vi "set_synth.vi"(0 "VISA resource name":refnum<visa-resource-name>, 1 "wfm?":bool, 3 "Arbitrary Waveform Name (\"ARB1\")":string="ARB1", 5 "Tot Synth Arr":dbl[](array[numeric]), 7 "error in (no error)":errorcluster, 9 "Enable Output (T: Enable)":bool=TRUE, 11 "Arbitrary Waveform Data":dbl[](array[numeric]), 12 "Trigger Synth":bool, 14 "Burst Count":i32=1) -> (4 "VISA resource name out":refnum<visa-resource-name>, 15 "error out":errorcluster)   [LabVIEW 2016]
uses:
  <instrlib>/Agilent 33XXX Series/Agilent 33XXX Series.lvlib
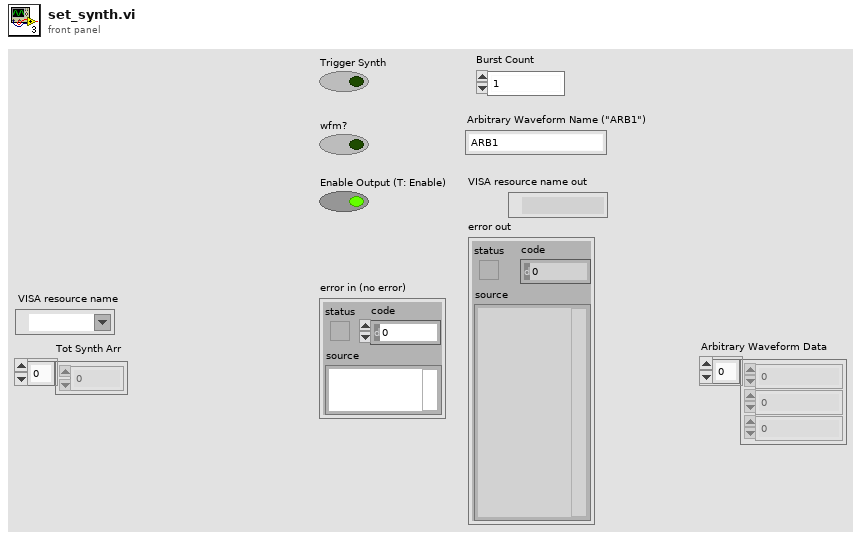
[diagram p1: front panel]
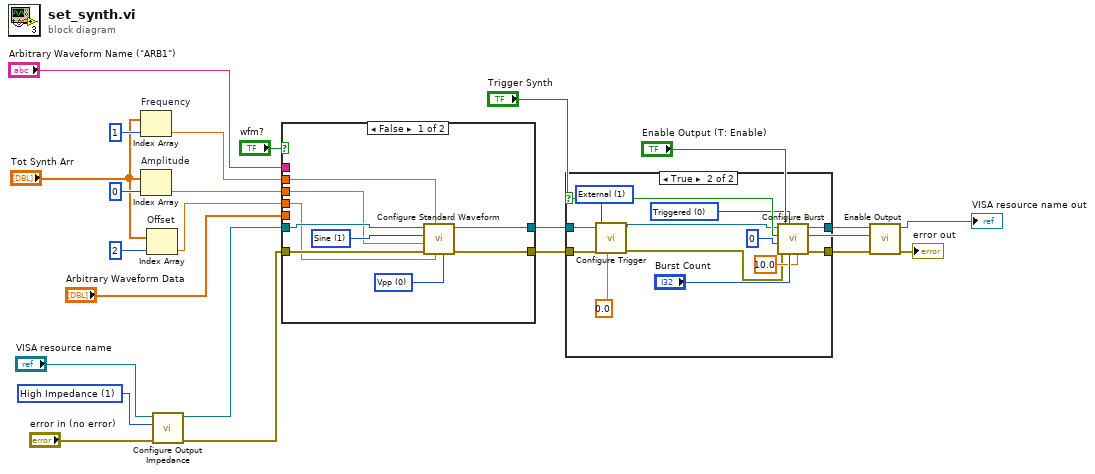
[diagram p0: block diagram]
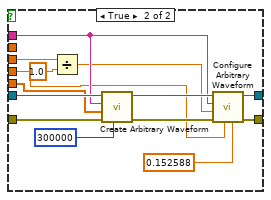
[diagram p3: hidden frame]
diagram:
  w13 = u16 1 items=["50 Ohms", "High Impedance", "User Defined"] ("Impedance (0: 50 Ohms)")
  n1 = Index Array "Frequency"(array="Tot Synth Arr", index=1) -> (element=w20:dbl)
  n2 = Index Array "Amplitude"(array="Tot Synth Arr", index=0) -> (element=w18:dbl)
  n3 = Index Array "Offset"(array="Tot Synth Arr", index=2) -> (element=w15:dbl)
  n4 = call <instrlib>:"Configure Output Impedance.vi"("error in (no error)"="error in (no error)", "Impedance (0: 50 Ohms)"=w13, "VISA resource name"="VISA resource name") -> ("error out"=w22:errorcluster, "VISA resource name out"=w23:refnum<visa-resource-name>)  [unwired: 7 in]
  n5 = case shown="False" "wfm?" {
    tunnel: w23 -> [w30 w41]
    tunnel: w22 -> [w29 w43]
    tunnel: w20 -> [w28 _]
    tunnel: w18 -> [w27 w36]
    tunnel: w15 -> [w26 w33]
    tunnel: [w25 w46] -> w5
    tunnel: [w24 w45] -> w3
    tunnel: "Arbitrary Waveform Name (\"ARB1\")" -> [_ w39]
    tunnel: "Arbitrary Waveform Data" -> [_ w38]
    frame False {
      w31 = u16 0 items=["Vpp", "Vrms", "dB"] ("Unit (0: Vpp)")
      w32 = u16 1 items=["DC", "Sine", "Square", "Triangle", "Ramp", "Pulse", "Noise", "Sinc", "Negative Ramp", "Exponential Rise", "Exponential Fall", "Cardiac"] ("Waveform Function (1: Sine)")
      n6 = call <instrlib>:"Configure Standard Waveform.vi"("Unit (0: Vpp)"=w31, "DC Offset (0.00 V)"=w26, "Frequency (1000 Hz)"=w28, "error in (no error)"=w29, "Amplitude (1)"=w27, "Waveform Function (1: Sine)"=w32, "VISA resource name"=w30) -> ("error out"=w24:errorcluster, "VISA resource name out"=w25:refnum<visa-resource-name>)  [unwired: 3 in]
    }
    frame True {
      n7 = Divide(x=w36, y=1.0) -> (x/y=w35:dbl)
      n8 = call <instrlib>:"Create Arbitrary Waveform.vi"("Timeout (10000)"=300000, "error in (no error)"=w43, "Arbitrary Waveform Data"=w38, "Arbitrary Waveform Name (\"ARB1\")"=w39, "VISA resource name"=w41) -> ("error out"=w42:errorcluster, "VISA resource name out"=w40:refnum<visa-resource-name>)  [unwired: 5 in]
      n9 = call <instrlib>:"Configure Arbitrary Waveform.vi"("Frequency (1000 Hz)"=0.152588, "Offset (0.00 V)"=w33, "error in (no error)"=w42, "Gain (1.0)"=w35, "Arbitrary Waveform Name (\"ARB1\")"=w39, "VISA resource name"=w40) -> ("error out"=w45:errorcluster, "VISA resource name out"=w46:refnum<visa-resource-name>)  [unwired: 4 in]
    }
  }
  n10 = case shown="True" "Trigger Synth" {
    selector: "Trigger Synth" -> [_ w61]
    tunnel: w5 -> [w48 w54]
    tunnel: [w48 w60] -> w4
    tunnel: w3 -> [w47 w52]
    tunnel: [w47 w59] -> w2
    frame False {
    }
    frame True {
      w49 = u16 1 items=["Internal", "External", "Software (bus)"] ("Trigger Source (0: Internal)")
      w58 = u16 0 items=["Triggered", "Gated"] ("Burst Mode (0: Triggered)")
      n11 = call <instrlib>:"Configure Trigger.vi"("Delay (0.0 s)"=0.0, "error in (no error)"=w52, "Trigger Source (0: Internal)"=w49, "VISA resource name"=w54) -> ("error out"=w51:errorcluster, "VISA resource name out"=w53:refnum<visa-resource-name>)  [unwired: 6 in]
      n12 = call <instrlib>:"Configure Burst.vi"("Burst Period (1 s)"=10.0, "Burst Count (1)"="Burst Count", "Burst Mode (0: Triggered)"=w58, "error in (no error)"=w51, "Burst Phase (0 deg)"=0, "Enable Burst (T: Enable)"=w61, "VISA resource name"=w53) -> ("error out"=w59:errorcluster, "VISA resource name out"=w60:refnum<visa-resource-name>)  [unwired: 3 in]
    }
  }
  n13 = call <instrlib>:"Enable Output.vi"("error in (no error)"=w2, "Enable Output  (T: Enable)"="Enable Output (T: Enable)", "VISA resource name"=w4) -> ("error out"=→"error out":errorcluster, "VISA resource name out"=→"VISA resource name out":refnum<visa-resource-name>)  [unwired: 7 in]
